vi "ROS_Topic_Read_Wait.vi"(2 "Timeout (ms)":i32=3000, 3 "ROS in":T1) -> (0 "Reply":string, 1 "ROS out":T1)   [LabVIEW 2013]
doc: "Waits for a non-empty message on the ROS topic or service until Timeout."
uses:
  SubVIs/_ROSControl.ctl
  SubVIs/_ROSDirection.ctl
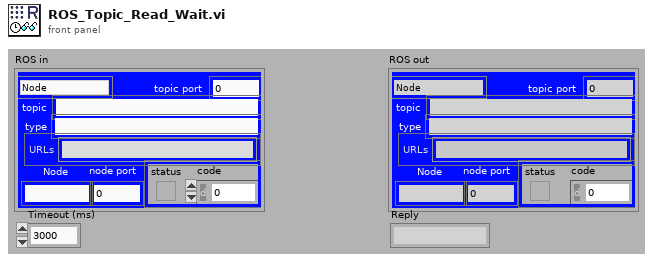
[diagram p1: front panel]
types:
  T1 = typedef "_ROSControl.ctl" = cluster{"topic port":u16, "Node":string, "topic":string, "type":string, "node port":u32, "error ":errorcluster, "Direction":T2, "APIs":string[]}
  T2 = typedef "_ROSDirection.ctl" = enum16{"Node", "Publisher", "Subscriber", "Service Client"}
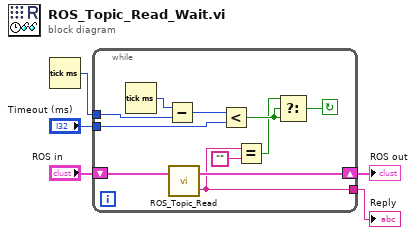
[diagram p0: block diagram]
diagram:
  n1 = Tick Count (ms)() -> (millisecond timer value=w1:u32)
  n2 = while {
    shift-right: [w15] -> w4
    shift-left: "ROS in" -> [w14]
    tunnel: [w13] -> w3
    tunnel: "Timeout (ms)" -> [w9]
    tunnel: w1 -> [w11]
    stop <- w6 continue-if-true
    n3 = Tick Count (ms)() -> (millisecond timer value=w12:u32)
    n4 = Subtract(x=w12, y=w11) -> (x-y=w10:u32)
    n5 = call "ROS_Topic_Read.vi"("ROS in"=w14) -> ("Reply"=w13:string, "ROS out"=w15:T1)  [unwired: 1 in]
    n6 = Less?(x=w10, y=w9) -> (x < y?=w8:bool)
    n7 = Equal?(x=w13, y="") -> (x = y?=w7:bool)
    n8 = Select(t=w7, s=w8, f=w8) -> (s? t:f=w6:bool)
  }
  "ROS out" <- w4
  "Reply" <- w3
